vi "Save_Waveforms.vi"(7 "Cluster":T1 {"File Location" items=["Unknown"=-1, "Processing"=0, "Storage"=1]; "Estimate Source" items=["Any Source."=-2, "No Shot"=-1, "Basic Labview Estimate"=0, "IDL Estimate From Andrew"=1, "IDL Estimate From Tobin"=2, "Old Metadata"=3]}, 8 "error in (no error)":errorcluster, 10 "id_dust_event":i64, 11 "ref":i32) -> (0 "error out":errorcluster, 3 "ref out":i32)   [LabVIEW 2013]
uses:
  Public API/Query_Dust_Event.ctl
  Controls/Estimate_source.ctl
  Controls/File_location.ctl
  <vilib>/addons/h5labview/H5F_mode.ctl
  <userlib>/_OpenG.lib/file/file.llb/File Exists - Scalar__ogtk.vi
  <vilib>/addons/h5labview/H5File.lvlib
  <vilib>/addons/h5labview/H5GroupObject.lvlib
panel:
  # "Dust Event"
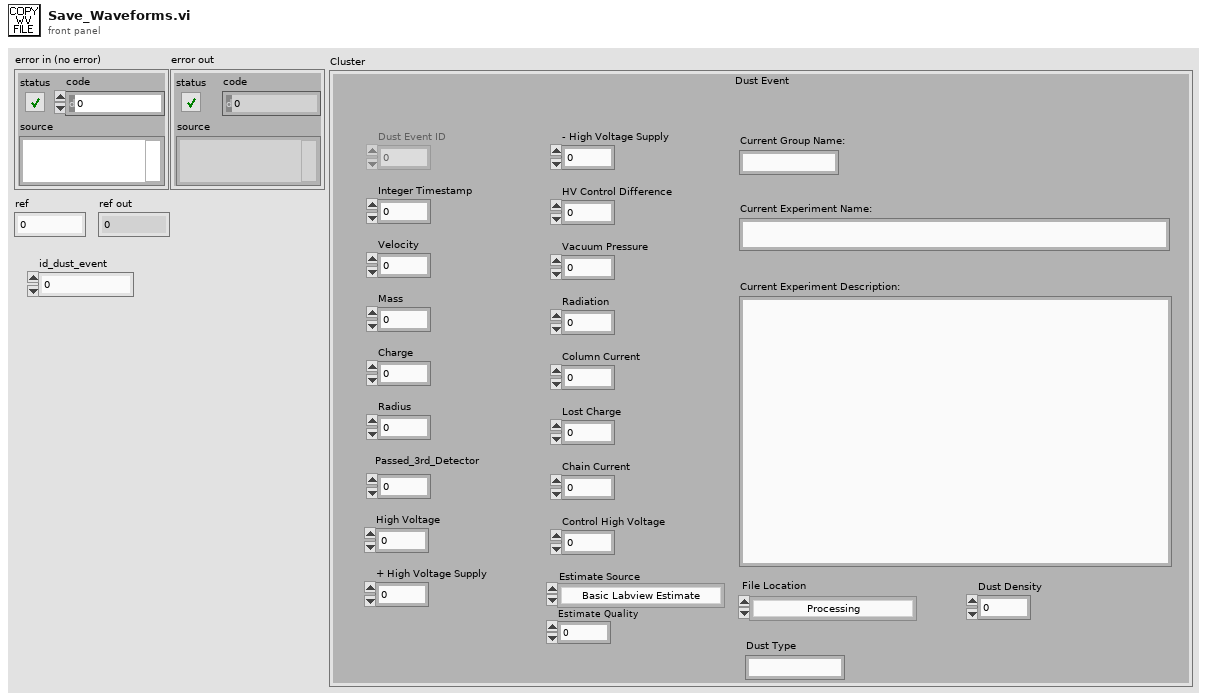
[diagram p1: front panel]
types:
  T1 = typedef "Query_Dust_Event.ctl" = cluster{"Dust Event ID":i64, "Integer Timestamp":i64, "Velocity":sgl, "Mass":sgl, "Charge":sgl, "Radius":sgl, "Passed_3rd_Detector":i8, "High Voltage":sgl, "+ High Voltage Supply":sgl, "- High Voltage Supply":sgl, "HV Control Difference":sgl, "Vacuum Pressure":sgl, "Radiation":sgl, "Column Current":sgl, "Lost Charge":sgl, "Chain Current":sgl, "Control High Voltage":sgl, "Current Group Name:":string, "Current Experiment Name:":string, "Current Experiment Description:":string, "Estimate Source":T2, "Estimate Quality":i8, "File Location":T3, "Dust Type":string, "Dust Density":sgl}
  T2 = typedef "Estimate_source.ctl" = i8
  T3 = typedef "File_location.ctl" = i8
  T4 = typedef "H5File.lvlib/H5F_mode.ctl" = enum16{"read-only", "read-write", "overwrite", "create new", "open or create"}
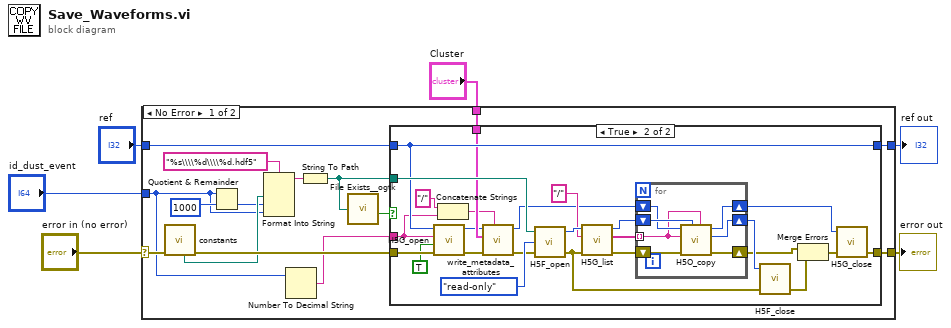
[diagram p0: block diagram]
diagram:
  n1 = case shown="No Error" "error in (no error)" {
    selector: "error in (no error)" -> [w15 w57]
    tunnel: [w12 w57] -> w4
    tunnel: "id_dust_event" -> [w11 _]
    tunnel: "ref" -> [w9 w56]
    tunnel: [w8 w56] -> w2
    tunnel: "Cluster" -> [w7 _]
    frame No Error {
      n2 = call "constants.vi"("error in (no error)"=w15) -> ("error out"=w21:errorcluster, "file path for Processed Signal .hdf5 files"=w18:path)  [unwired: 5 in, 4 out]
      n3 = Quotient & Remainder(x=w11, y=i64 1000) -> (floor(x/y)=w17:i64)  [unwired: 1 out]
      n4 = Format Into String(format string="%s\\\\%d\\\\%d.hdf5", w18, w17, w11) -> (resulting string=w16:string)  [unwired: 2 in, 1 out]
      n5 = Number To Decimal String(number=w11) -> (decimal integer string=w10:string)  [unwired: 1 in]
      n6 = String To Path(string=w16) -> (path=w14:path)
      n7 = call-poly <userlib>:"File Exists__ogtk.vi"("file path"=w14) -> ("exists"=w13:bool)  [unwired: 6 in, 1 out]
      n8 = case shown="True" w13 {
        tunnel: w21 -> [w23 w40]
        tunnel: w14 -> [_ w47]
        tunnel: [w23 w38] -> w12
        tunnel: w9 -> [w22 w32]
        tunnel: [w22 w32] -> w8
        tunnel: w10 -> [_ w27]
        tunnel: w7 -> [_ w29]
        frame False {
        }
        frame True {
          n9 = call <vilib>:"H5G_open.vi"("error in (no error)"=w40, "create? (F)"=TRUE, "name"=w27, "ref"=w32) -> ("error out"=w31:errorcluster, "group"=w28:i32)  [unwired: 2 in]
          n10 = Concatenate Strings("/" ("string"), w27) -> (w25:string)
          n11 = call "write_metadata_attributes.vi"("Group ID"=w25, "error in (no error)"=w31, "Cluster"=w29, "group ref"=w28) -> ("error out"=w30:errorcluster, "group ref out"=w26:i32)  [unwired: 4 in]
          n12 = call <vilib>:"H5F_open.vi"("error in (no error)"=w30, "mode"=H5F_mode."read-only", "path"=w47) -> ("error out"=w36:errorcluster, "ref"=w46:i32)  [unwired: 1 in]
          n13 = call <vilib>:"H5G_list.vi"("error in (no error)"=w36, "group"="/", "ref"=w46) -> ("error out"=w45:errorcluster, "names"=w43:string[], "ref out"=w44:i32)  [unwired: 1 in, 1 out]
          n14 = for {
            shift-right: [w52] -> w33
            shift-left: w45 -> [w55]
            shift-right: [w53] -> w42
            shift-left: w44 -> [w54]
            tunnel: w43 -> [w49] mode=indexing
            shift-right: [w50] -> w37
            shift-left: w26 -> [w51]
            n15 = call <vilib>:"H5O_copy.vi"("src_name"=w49, "src_id"=w54, "error in (no error)"=w55, "dest_name"=w49, "dest_id"=w51) -> ("error out"=w52:errorcluster, "src out"=w53:i32, "dest out"=w50:i32)  [unwired: 4 in]
          }
          n16 = call <vilib>:"H5F_close.vi"("error in (no error)"=w36, "ref"=w42) -> ("error out"=w34:errorcluster)  [unwired: 3 in]
          n17 = Merge Errors(w33, w34) -> (w35:errorcluster)
          n18 = call <vilib>:"H5G_close.vi"("error in (no error)"=w35, "ref"=w37) -> ("error out"=w38:errorcluster)  [unwired: 3 in]
        }
      }
    }
    frame Error {
    }
  }
  "error out" <- w4
  "ref out" <- w2
